vi "DisabledPage.vi"(0 "TabCtl Refnum":refnum<vi>, 1 "FindHome?":bool) -> ()   [LabVIEW 2011]
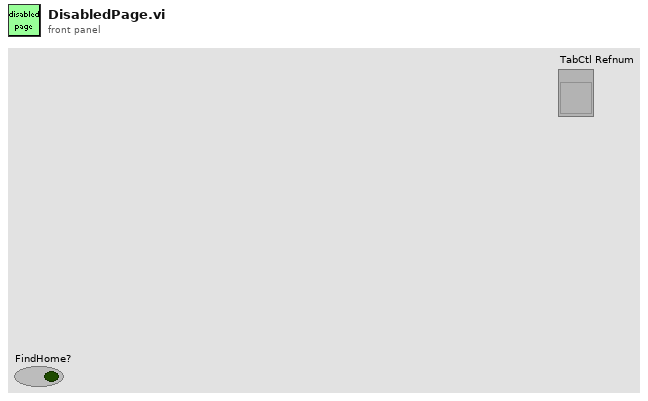
[diagram p1: front panel]
types:
  T1 = enum32{"Auto", "Error", "¦øªA¶b§ä­ìÂI", "³W®æ°Ñ¼Æ³]©w", "¬Û¾÷¹wÄý&¼v¹³¤ÀªR", "ÅJÀJ¯¸", "Other"}
  T2 = enum32{"Page Enabled", "Page Disabled", "Page Disabled & Grayed"}
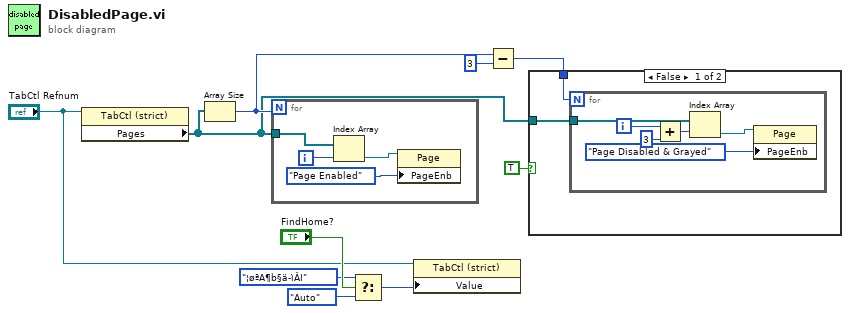
[diagram p0: block diagram]
diagram:
  n1 = property class="TabCtl (strict)"(reference="TabCtl Refnum") -> ("Pages"=w7:refnum<vi>[])  [unwired: 1 in, 2 out]
  n2 = Array Size(array=w7) -> (size(s)=w10:i32)
  n3 = for {
    N: w10 -> [_]
    tunnel: w7 -> [w12]
    i -> [w11]
    n4 = Index Array(array=w12, index=w11) -> (element=w14:refnum<vi>)
    n5 = property class="Page"(reference=w14, "PageEnb"=T2."Page Enabled" ("Page Enabled State")) -> ()  [unwired: 1 in, 2 out]
  }
  n6 = Select(t=T1."¦øªA¶b§ä­ìÂI", s="FindHome?", f=T1."Auto" ("Value")) -> (s? t:f=w2:T1)
  n7 = property on="Property Node" class="TabCtl (strict)"(reference="TabCtl Refnum", "Value"=w2) -> ()  [unwired: 1 in, 2 out]
  n8 = Subtract(x=w10, y=3) -> (x-y=w8:i32)
  n9 = case shown="False" TRUE {
    tunnel: w7 -> [w16 _]
    tunnel: w8 -> [w15 _]
    frame False {
      n10 = for {
        N: w15 -> [_]
        tunnel: w16 -> [w20]
        i -> [w18]
        n11 = Add(x=w18, y=3) -> (x+y=w19:i32)
        n12 = Index Array(array=w20, index=w19) -> (element=w22:refnum<vi>)
        n13 = property class="Page"(reference=w22, "PageEnb"=T2."Page Disabled & Grayed" ("Page Enabled State")) -> ()  [unwired: 1 in, 2 out]
      }
    }
    frame True {
    }
  }
